vi "Modified File Dialog.vi"(0 "start path":path=path "", 1 "prompt":string, 3 "button label":string, 7 "suggested filename":string, 11 "error in (no error)":errorcluster, 12 "pattern":string, 14 "pattern label":string) -> (4 "selected path":path, 8 "File exists":bool, 10 "Cancelled":bool, 15 "error out":errorcluster)   [LabVIEW 2019]
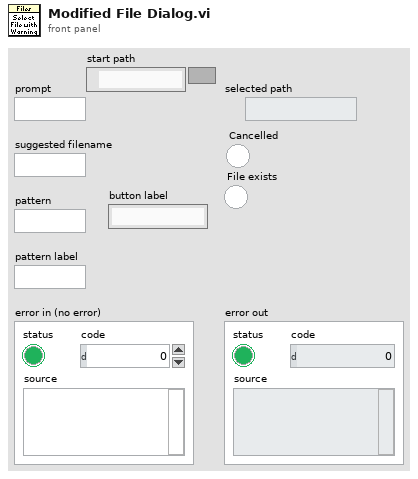
[diagram p1: front panel]
types:
  T1 = cluster{"Left Button Key Shortcut":cluster{"Control":bool, "Shift":bool, "Key":string}, "Center Button Key Shortcut":cluster{"Control":bool, "Shift":bool, "Key":string}, "Right Button Key Shortcut":cluster{"Control":bool, "Shift":bool, "Key":string}}
  T2 = enum16{"Left Button", "Center Button", "Right Button", "Window Close"}
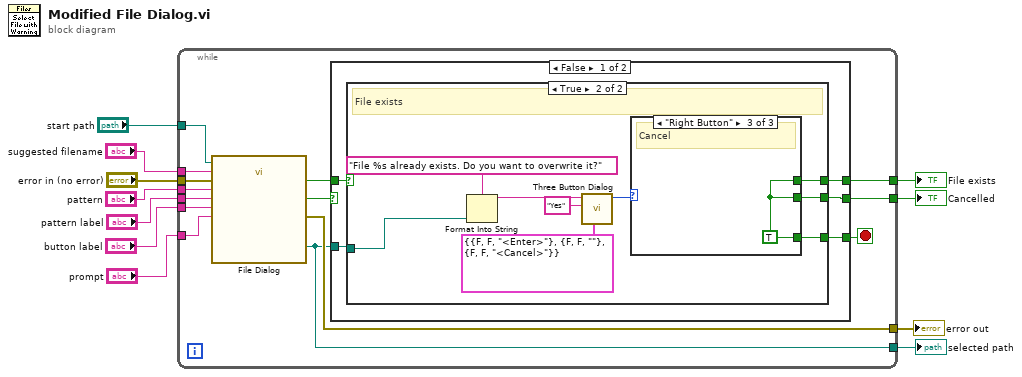
[diagram p0: block diagram]
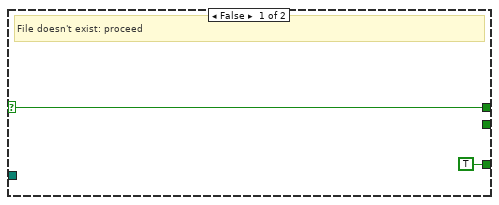
[diagram p2: hidden frame]
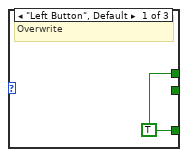
[diagram p3: hidden frame]
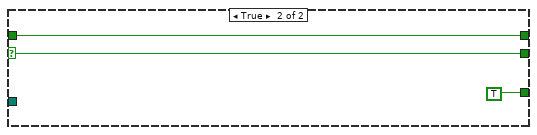
[diagram p5: hidden frame]
diagram:
  n1 = while {
    tunnel: "suggested filename" -> [w25]
    tunnel: "prompt" -> [w23]
    tunnel: "pattern" -> [w22]
    tunnel: "pattern label" -> [w21]
    tunnel: [w18] -> w6
    tunnel: "error in (no error)" -> [w24]
    tunnel: [w20] -> w5
    tunnel: [w16] -> w4
    tunnel: [w15] -> w3
    tunnel: "start path" -> [w13]
    tunnel: "button label" -> [w12]
    stop <- w17 stop-if-true
    n2 = call "File Dialog"("start path"=w13, "prompt"=w23, "button label"=w12, "default name"=w25, "error in"=w24, "pattern (all files)"=w22, "pattern label"=w21) -> ("selected path"=w18:path, "exists"=w19:bool, "cancelled"=w14:bool, "error out"=w20:errorcluster)  [unwired: 5 in]
    n3 = case shown="False" w14 {
      selector: w14 -> [_ w46]
      tunnel: w19 -> [w30 w45]
      tunnel: w18 -> [w29 _]
      tunnel: [w28 TRUE] -> w17
      tunnel: [w27 w45] -> w16
      tunnel: [w26 w46] -> w15
      frame False {
        n4 = case shown="True" w30 {
          selector: w30 -> [w31 _]
          tunnel: w29 -> [_ w36]
          tunnel: [TRUE w35] -> w28
          tunnel: [w31 w34] -> w27
          tunnel: [_ w33] -> w26
          frame False {
            # "File doesn't exist: proceed"
          }
          frame True {
            # "File exists"
            n5 = Format Into String(format string="File %s already exists. Do you want to overwrite it?", w36) -> (resulting string=w38:string)  [unwired: 2 in, 1 out]
            n6 = call <vilib>:"Three Button Dialog.vi"("Keyboard Shortcuts (Left is <Enter>)"=T1 {"Left Button Key Shortcut"={"Control"=FALSE, "Shift"=FALSE, "Key"="<Enter>"}, "Center Button Key Shortcut"={"Control"=FALSE, "Shift"=FALSE, "Key"=""}, "Right Button Key Shortcut"={"Control"=FALSE, "Shift"=FALSE, "Key"="<Cancel>"}}, "Left Button Text (\"Yes\")"="Yes" ("T button name (\"OK\")"), "message"=w38) -> ("Which Button?"=w40:T2)  [unwired: 8 in]
            n7 = case shown="\"Right Button\"" w40 {
              tunnel: [w42 _ w43] -> w35
              tunnel: [w42 _ w43] -> w34
              tunnel: [_ _ w43] -> w33
              frame "Left Button", Default {
                w42 = TRUE
                # "Overwrite"
              }
              frame "Center Button" {
                # "Try again"
              }
              frame "Right Button" {
                w43 = TRUE
                # "Cancel"
              }
            }
          }
        }
      }
      frame True {
      }
    }
  }
  "error out" <- w5
  "selected path" <- w6
  "File exists" <- w4
  "Cancelled" <- w3
